vi "counterTool_23_S.vi"(0 "Counts":dbl, 2 "Zero":bool, 4 "Output Units":enum16{"Degrees", "Radians"}(ring)) -> (6 "Total Angle":dbl=72.0, 7 "Wrap Angle":dbl)   [LabVIEW 2022 SP3]
doc: "Voltage - Input voltage value\nDeg/Volt - Constant multiplier to convert input voltage to angular value\n\nTotal Angle - Current accumulated angle -Inf to Inf degrees\nWrap Angle - Current angle 0 to 360 degrees"
panel:
  out "Cycles":dbl
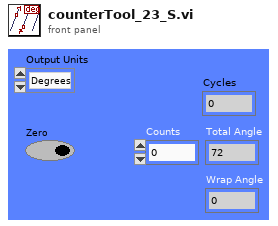
[diagram p1: front panel]
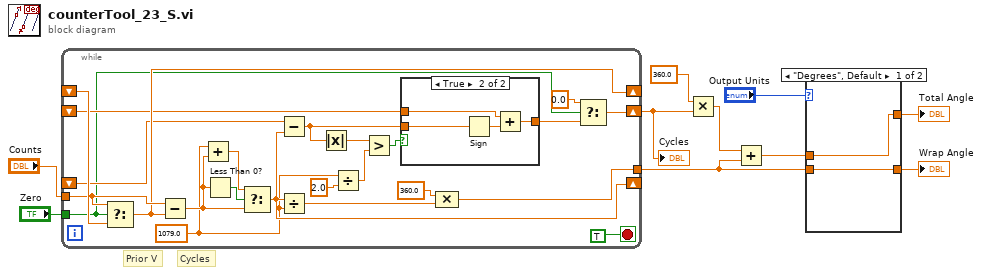
[diagram p0: block diagram]
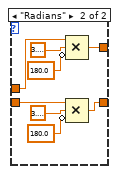
[diagram p2: hidden frame]
diagram:
  # "Prior V"
  # "Cycles"
  n1 = while {
    tunnel: [w23] -> w2
    shift-right: [w26] -> w9
    shift-left: _ -> [w15]
    tunnel: "Counts" -> [w21]
    shift-right: [w16] -> _
    shift-left: _ -> [w14]
    tunnel: "Zero" -> [w13]
    shift-right: [w20] -> _
    shift-left: _ -> [w22]
    stop <- TRUE stop-if-true
    w11 = 1079.0
    n2 = Select(t=w21, s=w13, f=w22) -> (s? t:f=w20:dbl)
    n3 = Subtract(x=w21, y=w20) -> (x-y=w17:dbl)
    n4 = Add(x=w11, y=w17) -> (x+y=w18:dbl)
    n5 = Less Than 0?(x=w17) -> (x < 0?=w19:bool)
    n6 = Select(t=w18, s=w19, f=w17) -> (s? t:f=w16:dbl)
    n7 = Subtract(x=w14, y=w16) -> (x-y=w30:dbl)
    n8 = Divide(x=w16, y=w11) -> (x/y=w27:dbl)
    n9 = Absolute Value(x=w30) -> (abs(x)=w32:dbl)
    n10 = Divide(x=w11, y=2.0) -> (x/y=w28:dbl)
    n11 = Greater?(x=w32, y=w28) -> (0:w31:bool)
    n12 = case shown="True" w31 {
      tunnel: [w34 w38] -> w25
      tunnel: w15 -> [w34 w37]
      tunnel: w30 -> [_ w36]
      frame False {
      }
      frame True {
        n13 = Sign(1:w36) -> (0:w35:dbl)
        n14 = Add(x=w37, y=w35) -> (x+y=w38:dbl)
      }
    }
    n15 = Compound Arithmetic op=MULTIPLY(360.0 ("y"), w27) -> (w23:dbl)
    n16 = Select(t=0.0, s=w13, f=w25) -> (s? t:f=w26:dbl)
  }
  "Cycles" <- w9
  n17 = Multiply(x=360.0 ("y"), y=w9) -> (x*y=w10:dbl)
  n18 = Add(x=w10, y=w2) -> (x+y=w4:dbl)
  n19 = case shown="\"Degrees\", Default" "Output Units" {
    tunnel: [w40 w46] -> w3
    tunnel: w4 -> [w40 w45]
    tunnel: w2 -> [w39 w42]
    tunnel: [w39 w41] -> w1
    frame "Degrees", Default {
    }
    frame "Radians" {
      n20 = Compound Arithmetic op=MULTIPLY(w45, 3.141592653589793, invert 180.0 ("value")) -> (w46:dbl)
      n21 = Compound Arithmetic op=MULTIPLY(w42, 3.141592653589793, invert 180.0 ("value")) -> (w41:dbl)
    }
  }
  "Wrap Angle" <- w1
  "Total Angle" <- w3
